vi "Socket Read.vi"(8 "error in (no error)":errorcluster, 9 "timeout ms (5000)":i32=5000, 10 "# bytes to read":i32, 11 "WebSocket in":refnum<class "WebSocket.lvclass">) -> (0 "error out":errorcluster, 2 "Read Bytes":u8[](array[numeric]), 3 "WebSocket out":refnum<class "WebSocket.lvclass">)   [LabVIEW 2013, in "WebSockets.lvlib" / "WebSocket.lvclass"]
uses:
  WebSocket.lvclass
  WebSocket.lvclass/WebSocket.ctl
  Sockets/Socket/Socket.lvclass
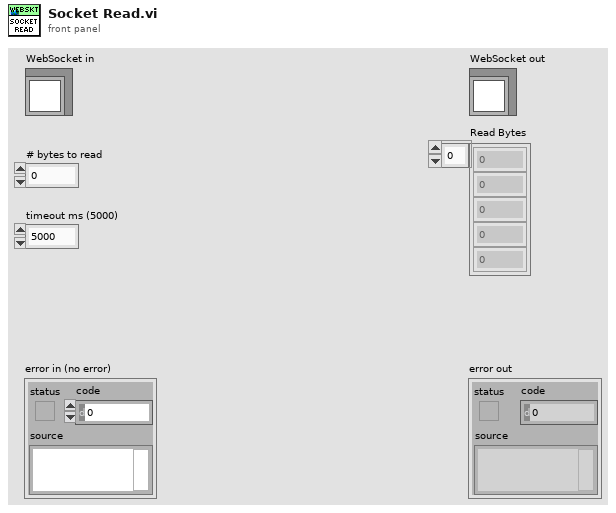
[diagram p1: front panel]
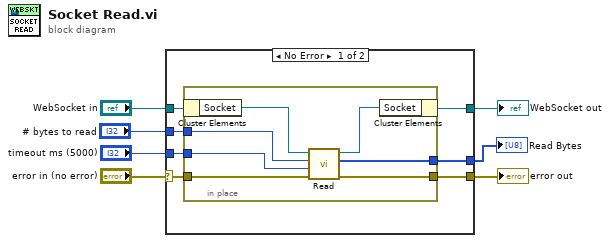
[diagram p0: block diagram]
diagram:
  n1 = case shown="No Error" "error in (no error)" {
    selector: "error in (no error)" -> [w12 w22]
    tunnel: [w10 w23] -> w5
    tunnel: "WebSocket in" -> [w14 w23]
    tunnel: "timeout ms (5000)" -> [w13 _]
    tunnel: [w11 w22] -> w3
    tunnel: [w9 _] -> w2
    tunnel: "# bytes to read" -> [w8 _]
    frame No Error {
      n2 = in-place {
        in-place-border: w13 -> [w20]
        in-place-border: w12 -> [w19]
        in-place-border: [w18] -> w11
        in-place-border: [w16] -> w9
        in-place-border: w8 -> [w15]
        n3 = in-place-cluster #1(w14) -> ("Socket"=w21:refnum<class "Socket.lvclass">)
        n4 = call-dynamic "Read.vi"("error in (no error)"=w19, "timeout ms (25000)"=w20, "# bytes to read"=w15, "Socket in"=w21) -> ("error out"=w18:errorcluster, "Read Bytes"=w16:u8[], "Socket out"=w17:refnum<class "Socket.lvclass">)  [unwired: 5 in]
        n5 = in-place-cluster #1("Socket"=w17) -> (w10:refnum<class "WebSocket.lvclass">)
      }
    }
    frame Error {
    }
  }
  "error out" <- w3
  "WebSocket out" <- w5
  "Read Bytes" <- w2
